vi "Check Display Trace.vi"(8 "Error In (no error)":errorcluster, 9 "Display Trace (1)":i32=1, 10 "Display Window (1)":i32=1, 11 "VISA Resource Name":refnum<visa-resource-name>) -> (0 "Error Out":errorcluster, 1 "Trace Array":i32[](array[numeric]), 2 "Display Trace Check":bool, 3 "VISA Resource Name Out":refnum<visa-resource-name>)   [LabVIEW 2018, in "Agilent PNA Series.lvlib"]
doc: "This VI checks that the display window number is valid for the selected channel."
uses:
  Agilent PNA Series.lvlib
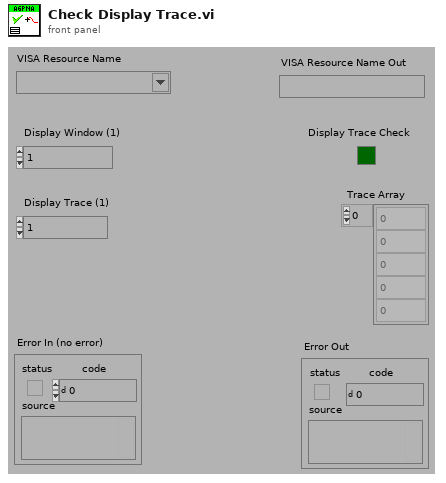
[diagram p1: front panel]
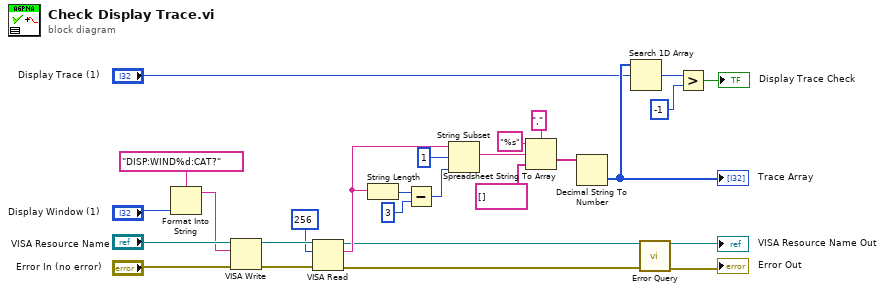
[diagram p0: block diagram]
diagram:
  n1 = Format Into String(format string="DISP:WIND%d:CAT?", "Display Window (1)") -> (resulting string=w5:string)  [unwired: 2 in, 1 out]
  n2 = VISA Write(VISA resource name="VISA Resource Name", write buffer=w5, error in (no error)="Error In (no error)") -> (VISA resource name out=w26:refnum<visa-resource-name>, error out=w25:errorcluster)  [unwired: 1 out]
  n3 = VISA Read(VISA resource name=w26, byte count=u32 256 ("byte count (0)"), error in (no error)=w25) -> (VISA resource name out=w4:refnum<visa-resource-name>, read buffer=w8:string, error out=w2:errorcluster)  [unwired: 1 out]
  n4 = String Length(string=w8) -> (length=w15:i32)
  n5 = Subtract(x=w15, y=3) -> (x-y=w13:i32)
  n6 = String Subset(string=w8, offset (0)=1, length (rest)=w13) -> (substring=w17:string)
  n7 = Spreadsheet String To Array(delimiter (Tab)=",", format string="%s", spreadsheet string=w17, array type (2D Dbl)=string[] []) -> (array=w12:string[])
  n8 = Decimal String To Number(string=w12) -> (number=w11:i32[])  [unwired: 2 in, 1 out]
  "Trace Array" <- w11
  n9 = Search 1D Array(1D array=w11, element="Display Trace (1)") -> (index of element=w10:i32)  [unwired: 1 in]
  n10 = call "Error Query.vi"("VISA Resource Name"=w4, "error in (no error)"=w2) -> ("VISA Resource Name Out"=→"VISA Resource Name Out":refnum<visa-resource-name>, "error out"=→"Error Out":errorcluster)  [unwired: 10 in, 2 out]
  n11 = Greater?(x=w10, y=-1) -> (0:→"Display Trace Check":bool)
